vi "DAC Save Results.vi"(8 "error in":errorcluster, 9 "Log Details?":bool, 10 "tdms file":refnum<k34>, 11 "DAC LN2 Temp in":refnum<class "DAC LN2 Temp.lvclass">) -> (0 "error out":errorcluster)   [LabVIEW 2019, in "DAC.lvlib" / "DAC LN2 Temp.lvclass"]
uses:
  DAC LN2 Temp.lvclass
  DAC.lvclass
  C:/Users/krio/Documents/LV_Projects/test-stand/App/DAC/DAC.lvclass
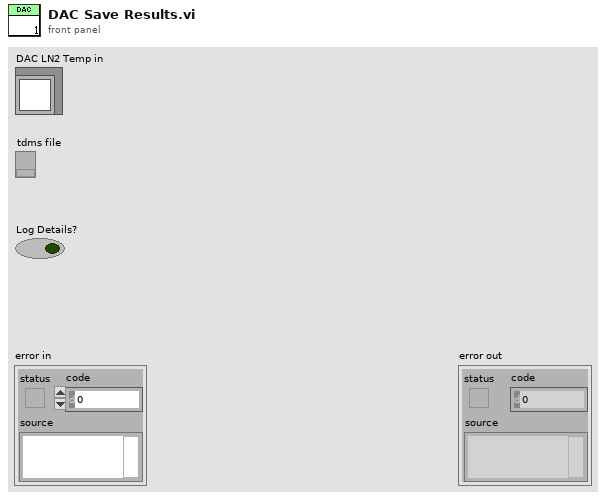
[diagram p1: front panel]
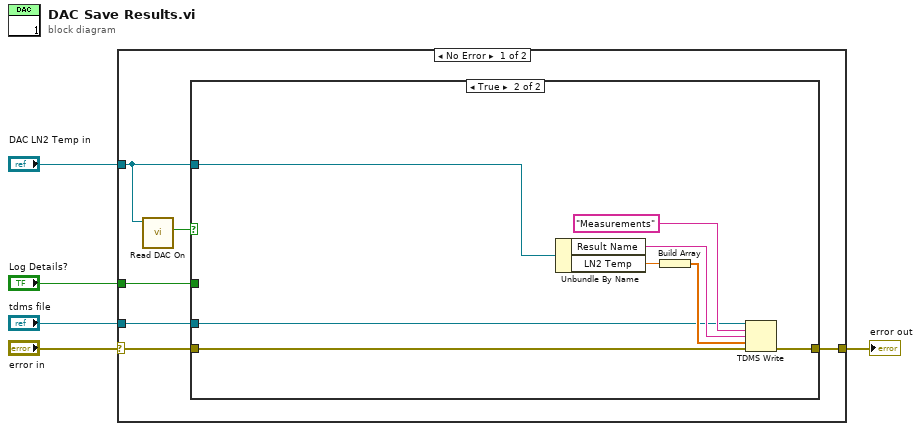
[diagram p0: block diagram]
diagram:
  n1 = case shown="No Error" "error in" {
    selector: "error in" -> [w8 w21]
    tunnel: "DAC LN2 Temp in" -> [w11 _]
    tunnel: "tdms file" -> [w9 _]
    tunnel: [w7 w21] -> w3
    tunnel: "Log Details?" -> [w6 _]
    frame No Error {
      n2 = call "Read DAC On.vi"("DAC in"=w11) -> ("DAC On"=w10:bool)  [unwired: 8 in, 2 out]
      n3 = case shown="True" w10 {
        tunnel: w11 -> [_ w16]
        tunnel: w9 -> [_ w14]
        tunnel: w8 -> [w12 w15]
        tunnel: [w12 w13] -> w7
        tunnel: w6 -> [_ _]
        frame False {
        }
        frame True {
          n4 = Unbundle By Name(w16) -> ("Result Name"=w18:string, "LN2 Temp"=w20:dbl)
          n5 = Build Array(w20) -> (w19:dbl[])
          n6 = TDMS Write(0:w14, 5:"Measurements" ("group name in (Untitled)"), 7:w18, 9:w19, 11:w15) -> (15:w13:errorcluster)  [unwired: 1 in, 3 out]
        }
      }
    }
    frame Error {
    }
  }
  "error out" <- w3
